vi "TRolly example.vi"() -> ()   [LabVIEW 2019]
uses:
  <vilib>/Rock Robotics/WPI/Joystick/WPI_JoystickArcadeMapping.vi
panel:
  in  "Trolly speed":dbl(slide)=0.44897959183673464 scale=0.0..1.0
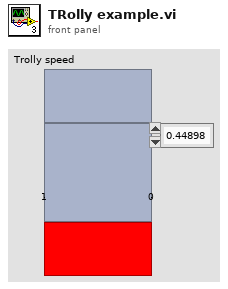
[diagram p1: front panel]
types:
  T1 = typedef "WPI_GyroDevRef.ctl" = cluster{"DevStatus":errorcluster, "Analog Channel":T2, "Gain (VoltsPerDegree/Second)":dbl, "Gyro Type":enum16{"Analog", "XRS450"}, "Handle":i32, "SPI Bus":T3, "Device Found":bool, "Sample Rate":dbl, "Calibrate On Open":bool, "Offset":dbl}
  T2 = typedef "FPGA_AIChannel.ctl" = enum8{"AI 0", "AI 1", "AI 2", "AI 3", "AI MXP 0", "AI MXP 1", "AI MXP 2", "AI MXP 3", "Invalid"}
  T3 = typedef "spi_bus.ctl" = enum16{"SPI On-Board, CS0", "SPI On-Board, CS1", "SPI On-Board, CS2", "SPI On-Board, CS3", "SPI MXP", "Invalid"}
  T4 = typedef "WPI_MotorControlDeviceRef.ctl" = cluster{"DeviceStatus":errorcluster, "Type":T5, "PWM":cluster{"PWM Channel":T6, "DeadBand":T7}, "CAN":cluster{"Device Number":u8, "SetOutput VI Ref":variant, "GetOutput VI Ref":variant, "Enable VI Ref":variant, "Disable VI Ref":variant, "Data":variant}, "Invert":bool, "DIO PWM":cluster{"PWM \"Enable\" Channel":T6, "DIOChannel":T8, "PWM Rate":dbl}}
  T5 = typedef "WPI_MotorControlType.ctl" = enum16{"PWM", "CAN", "DIO PWM"}
  T6 = typedef "FPGA_DIOPWMChannel.ctl" = enum8{"PWM 0", "PWM 1", "PWM 2", "PWM 3", "PWM 4", "PWM 5", "PWM 6", "PWM 7", "PWM 8", "PWM 9", "PWM MXP 0", "PWM MXP 1", "PWM MXP 2", "PWM MXP 3", "PWM MXP 4", "PWM MXP 5", "PWM MXP 6", "PWM MXP 7", "PWM MXP 8", "PWM MXP 9", "Invalid"}
  T7 = typedef "WPI_PWMDeadband.ctl" = cluster{"Name":string, "maxPositivePwm":i32, "minPositivePwm":i32, "centerPwm":i32, "maxNegativePwm":i32, "minNegativePwm":i32, "angularRange":u16}
  T8 = typedef "FPGA_DIOChannel.ctl" = enum8{"DIO 0", "DIO 1", "DIO 2", "DIO 3", "DIO 4", "DIO 5", "DIO 6", "DIO 7", "DIO 8", "DIO 9", "DIO MXP 0", "DIO MXP 1", "DIO MXP 2", "DIO MXP 3", "DIO MXP 4", "DIO MXP 5", "DIO MXP 6", "DIO MXP 7", "DIO MXP 8", "DIO MXP 9", "DIO MXP 10", "DIO MXP 11", "DIO MXP 12", "DIO MXP 13", "DIO MXP 14", "DIO MXP 15", "SPI Port CS1", "SPI Port CS2", "SPI Port CS3", "SPI Port MISO", "SPI Port MOSI", "Invalid"}
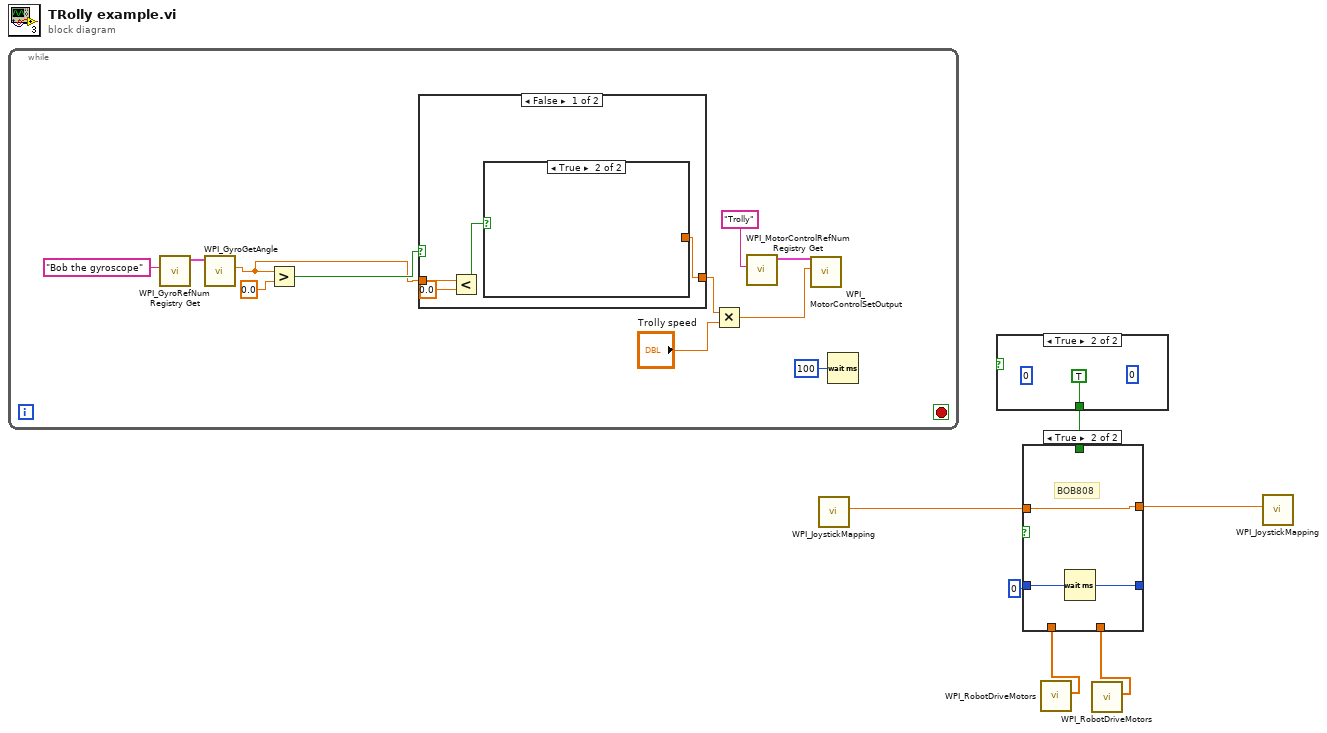
[diagram p0: block diagram]
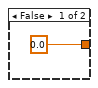
[diagram p2: hidden frame]
diagram:
  n1 = while {
    stop <- _ stop-if-true
    n2 = call <vilib>:"WPI_GyroRefNum Registry Get.vi"("refnum name"="Bob the gyroscope") -> ("GyroDevRef"=w11:T1)  [unwired: 9 in, 1 out]
    n3 = call <vilib>:"WPI_GyroGetAngle.vi"("GyroDevRef"=w11) -> ("Angle"=w8:dbl)  [unwired: 7 in, 3 out]
    n4 = Greater?(x=w8, y=0.0) -> (0:w9:bool)
    n5 = case shown="False" w9 {
      tunnel: w8 -> [w21 w23]
      tunnel: [w18 w23] -> w13
      frame False {
        n6 = Less?(x=w21, y=0.0) -> (x < y?=w19:bool)
        n7 = case shown="True" w19 {
          tunnel: [0.0 _] -> w18
          frame False {
          }
          frame True {
          }
        }
      }
      frame True {
      }
    }
    n8 = Multiply(x=w13, y="Trolly speed") -> (x*y=w15:dbl)
    n9 = call <vilib>:"WPI_MotorControlRefNum Registry Get.vi"("refnum name"="Trolly") -> ("MotorControlDevRef"=w17:T4)  [unwired: 9 in, 1 out]
    n10 = call <vilib>:"WPI_MotorControlSetOutput.vi"("Output"=w15, "MotorControlDevRef"=w17) -> ()  [unwired: 7 in, 3 out]
    n11 = Wait (ms)(milliseconds to wait=u32 100) -> ()  [unwired: 1 out]
  }
  n12 = call-poly <vilib>:"WPI_JoystickMapping.vi"() -> ("Left Motor Value"=w4:dbl)  [unwired: 10 in, 1 out]
  n13 = case shown="True" {
    selector: _ -> [_ _]
    tunnel: [_ TRUE] -> w6
    frame False {
    }
    frame True {
      (unwired) 0
      (unwired) 0
    }
  }
  n14 = call <vilib>:"WPI_RobotDriveMotors.vi"() -> ("Motor Values"=w3:dbl[])  [unwired: 9 in, 2 out]
  n15 = call <vilib>:"WPI_RobotDriveMotors.vi"() -> ("Motor Values"=w2:dbl[])  [unwired: 9 in, 2 out]
  n16 = case shown="True" {
    selector: _ -> [_ _]
    tunnel: w6 -> [_ _]
    tunnel: w4 -> [_ w27]
    tunnel: [_ w27] -> w5
    tunnel: w3 -> [_ _]
    tunnel: w2 -> [_ _]
    tunnel: 0 -> [_ w26]
    tunnel: [_ w25] -> _
    frame False {
    }
    frame True {
      # "BOB808"
      n17 = Wait (ms)(milliseconds to wait=w26) -> (millisecond timer value=w25:u32)
    }
  }
  n18 = call-poly <vilib>:"WPI_JoystickMapping.vi"("X axis value"=w5) -> ()  [unwired: 9 in, 2 out]
